vi "Get Data.vi"(8 "error in (no error)":errorcluster, 11 "Message in":refnum<class "Message.lvclass">) -> (0 "error out":errorcluster, 2 "Data":string, 3 "Message out":refnum<class "Message.lvclass">)   [LabVIEW 2020, in "Stream-Simple-Msg.lvlib" / "Message.lvclass"]
uses:
  Message.lvclass
  Message.lvclass/Message.ctl
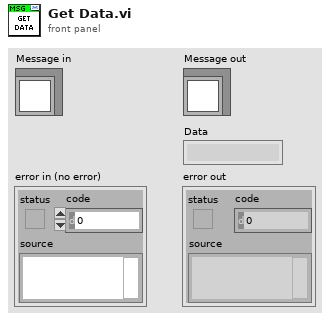
[diagram p1: front panel]
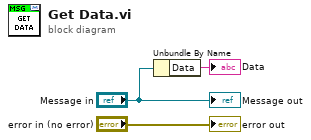
[diagram p0: block diagram]
diagram:
  n1 = Unbundle By Name("Message in") -> ("Data"=→"Data":string)
  "error out" <- "error in (no error)"
  "Message out" <- "Message in"
